vi "Untitled 1.vi"() -> ()   [LabVIEW 2020]
uses:
  <vilib>/Enthought/Python Integration Toolkit/api/Get Value String.vi
  <vilib>/Enthought/Python Integration Toolkit/Python Integration Toolkit.lvlib
panel:
  out "Value":string
  in  "Object Name":string
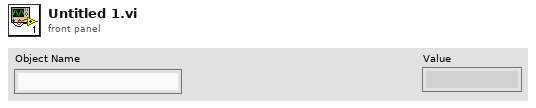
[diagram p1: front panel]
types:
  T1 = typedef "Python Integration Toolkit.lvlib/Session ID.ctl" = u64
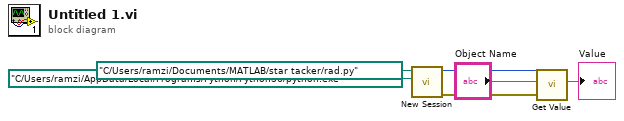
[diagram p0: block diagram]
diagram:
  n1 = call <vilib>:"New Session.vi"("Optional Path to Python.exe"=path "C:/Users/ramzi/AppData/Local/Programs/Python/Python36/python.exe", "Path to Python Module (.py File)"=path "C:/Users/ramzi/Documents/MATLAB/star tacker/rad.py") -> ("error out"=w3:errorcluster, "Session ID out"=w6:T1)  [unwired: 8 in]
  n2 = call-poly <vilib>:"Get Value.vi"("error in (no error)"=w3, "Object Name"="Object Name", "Session ID"=w6) -> ("Value"=→"Value":string)  [unwired: 6 in, 2 out]
